vi "Constants.vi"() -> ()   [LabVIEW 2019, in "Untitled Project 2 Shared.lvlib"]
doc: "Use this Global VI to access the GUIDs assigned to the page resources of the Custom Device."
uses:
  Untitled Project 2 Shared.lvlib
panel:
  in  "Tab Control":enum32{"GUIDS", "Constants", "Properties"}(tab)
  in  "test":string="a653e7e7-b07f-4a93-8843-5bf9e1db099a"
  in  "Untitled Project 2":string="9aec6653-8d94-44d4-9685-523138ab798f"
  in  "Compiled.Settings":string="Compiled.Settings"
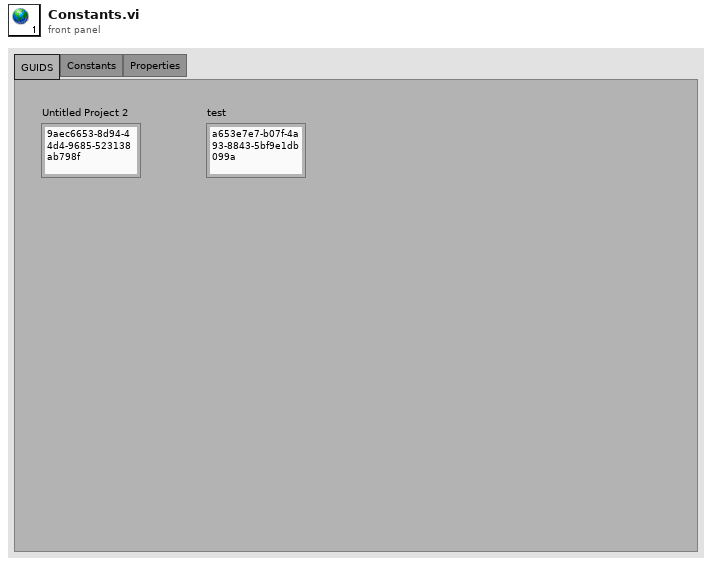
[diagram p1: front panel]
diagram:
